vi "Configure Dialog.vi"(8 "error in (no error)":errorcluster, 11 "Configure AM Internal [AM] Msg.lvclass":refnum<class "Configure AM Internal [AM] Msg.lvclass">) -> (0 "error out":errorcluster, 2 "Ok?":bool, 3 "Configure AM Internal [AM] Msg.lvclass":refnum<class "Configure AM Internal [AM] Msg.lvclass">)   [LabVIEW 2015, in "CS++Fgen.lvlib" / "Configure AM Internal [AM] Msg.lvclass"]
uses:
  Configure AM Internal [AM] Msg.lvclass
  Configure AM Internal [AM] Msg.lvclass/Configure AM Internal [AM] Msg.ctl
panel:
  in  "modulation waveform (Sine)":i32
  in  "Cancel Button":bool
  in  "OK Button":bool
  in  "modulation frequency":dbl[unit]
  in  "modulation depth":dbl
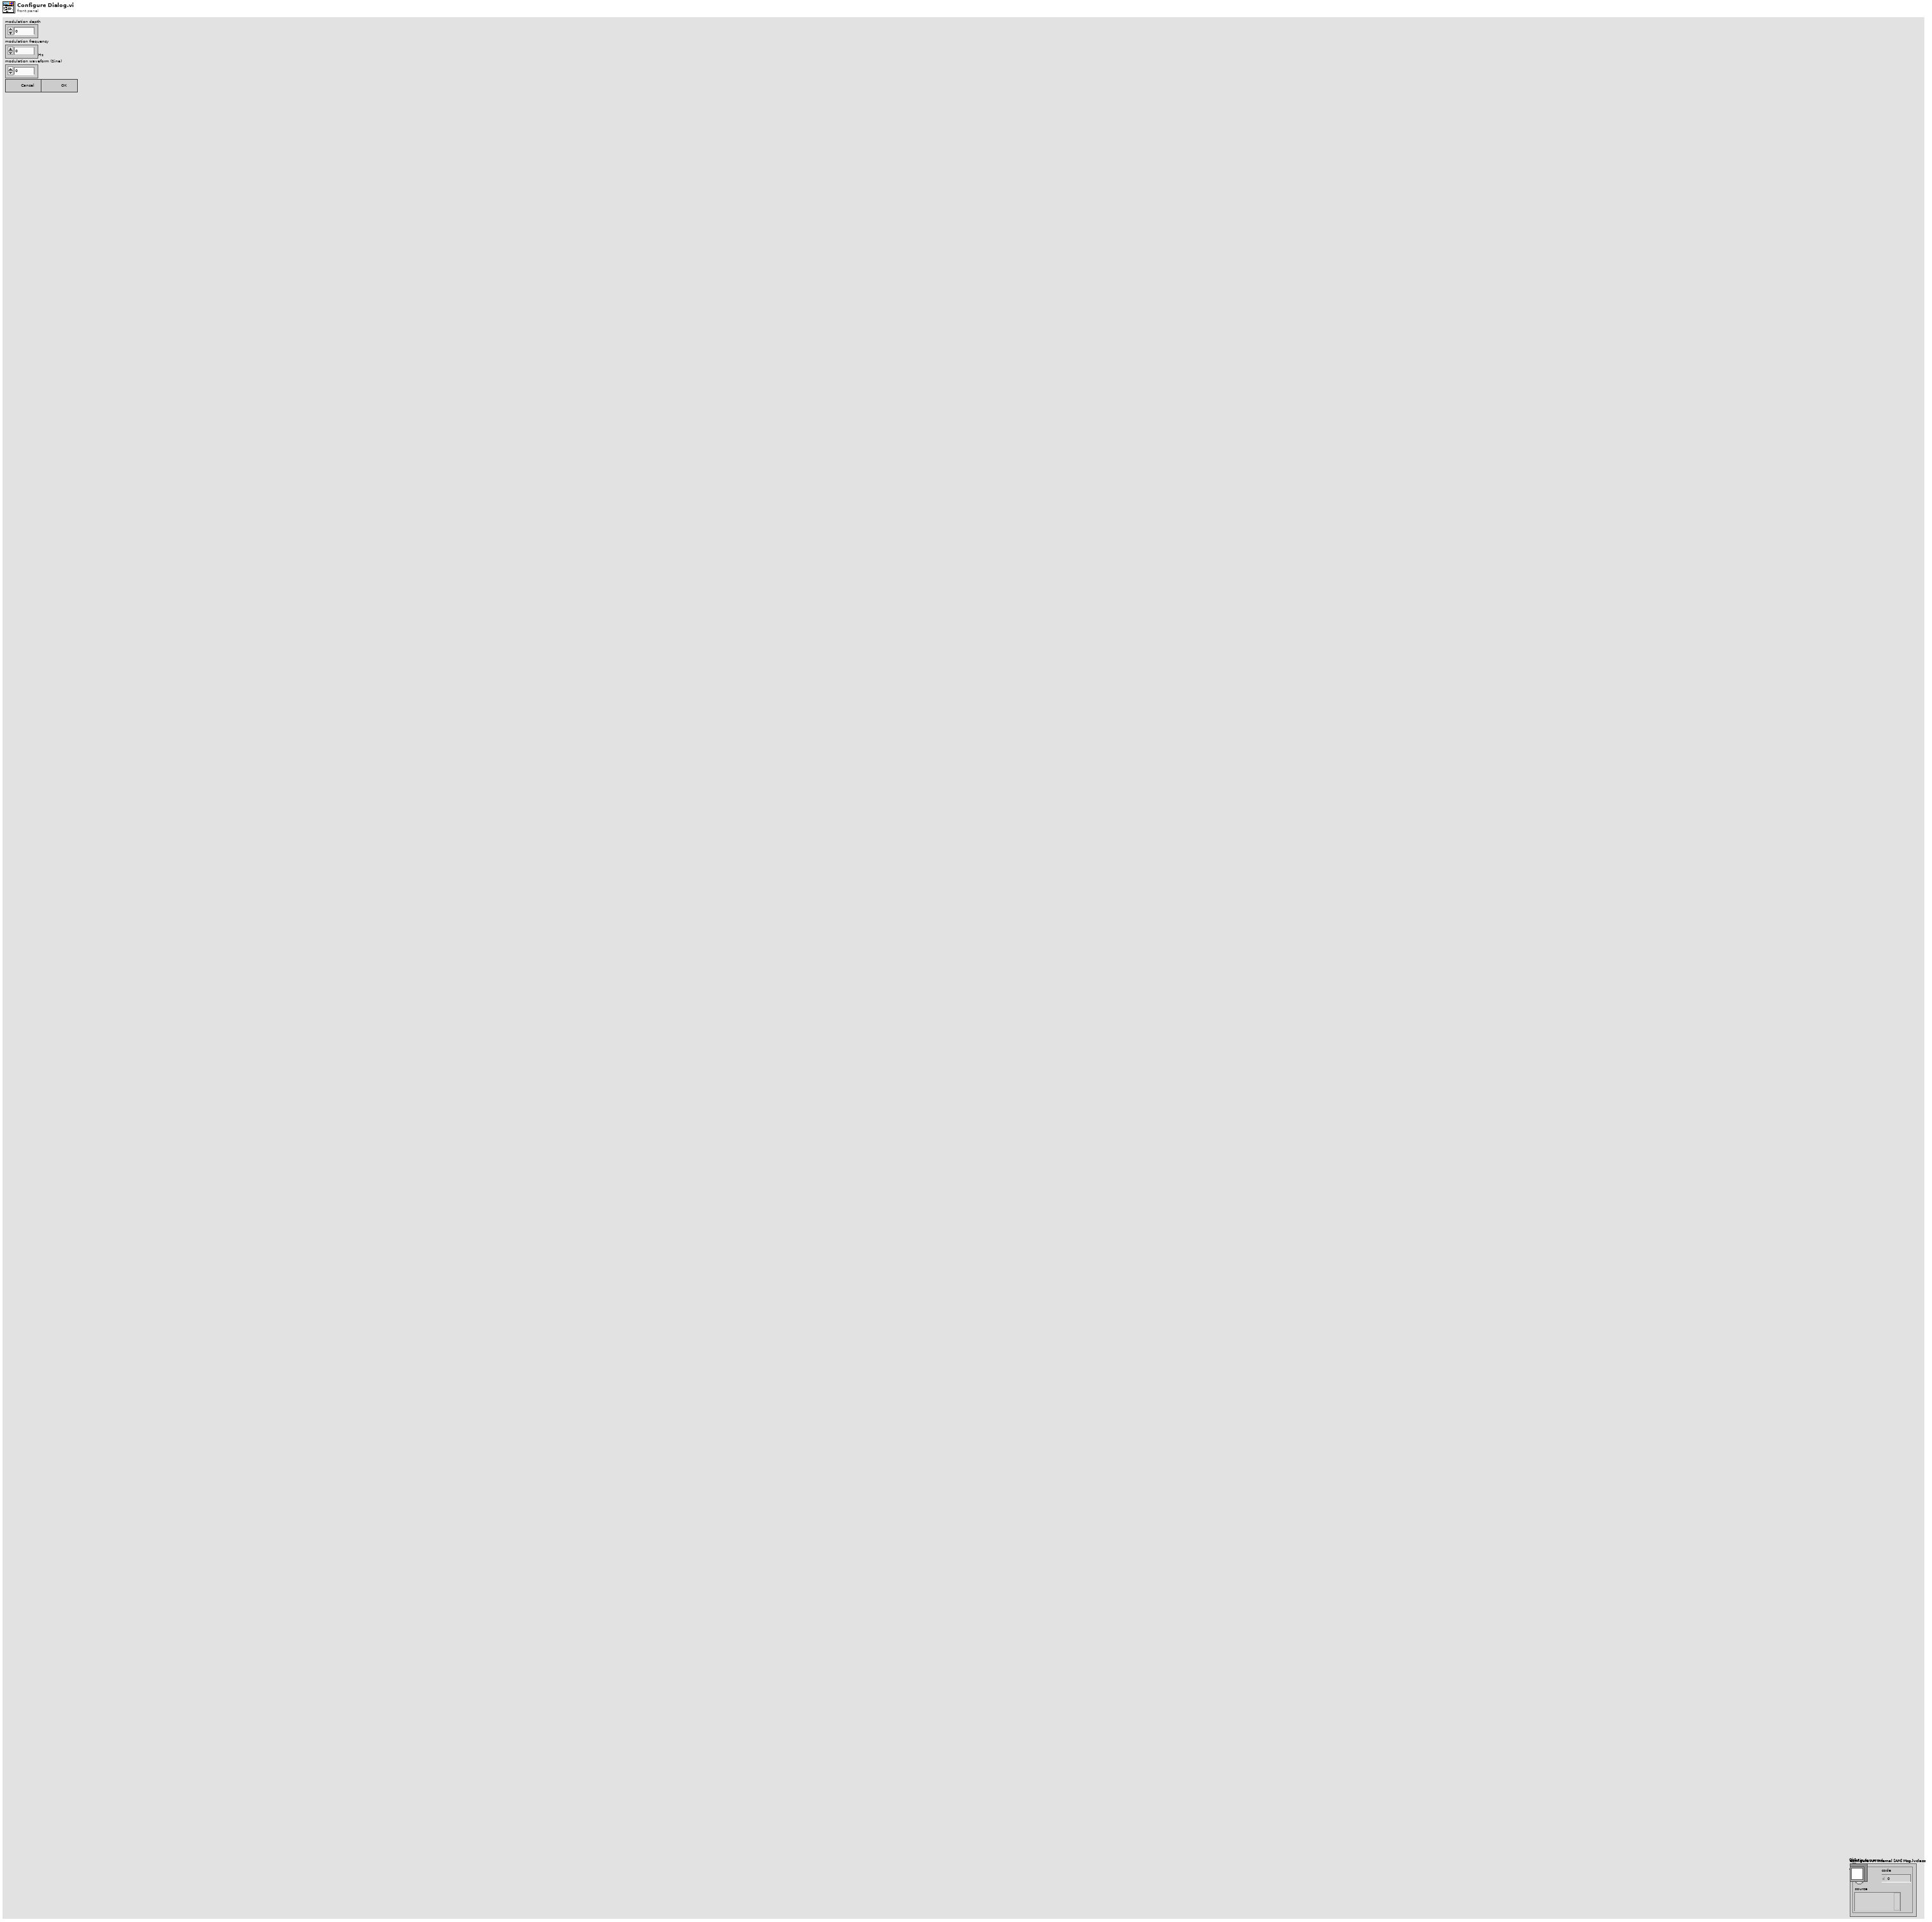
[diagram p1: front panel]
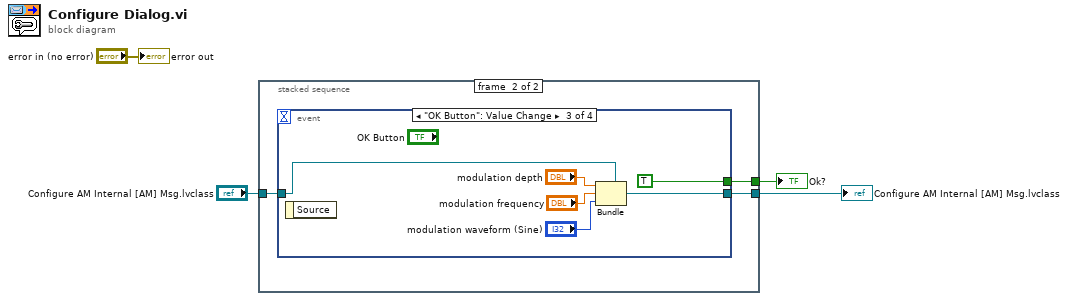
[diagram p0: block diagram]
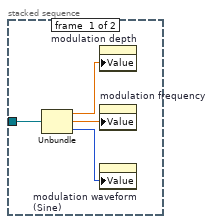
[diagram p2: hidden frame]
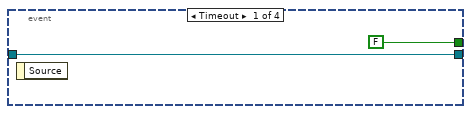
[diagram p3: hidden frame]
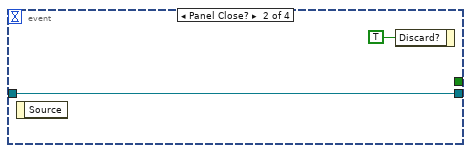
[diagram p4: hidden frame]
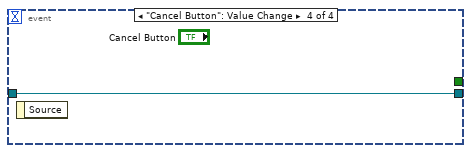
[diagram p5: hidden frame]
diagram:
  n1 = stacked-sequence {
    tunnel: [_ w11] -> w3
    tunnel: [_ w10] -> w2
    tunnel: "Configure AM Internal [AM] Msg.lvclass" -> [w8 w9]
    frame #0 {
      n2 = Unbundle ("Seq0Unbundler")(w8) -> (w7:dbl, w6:dbl[unit], w5:i32)
      n3 = property on="modulation depth" class="DigNum (strict)"("Value"=w7) -> ()  [unwired: 2 in, 2 out]
      n4 = property on="modulation frequency" class="DigNum (strict)"("Value"=w6) -> ()  [unwired: 2 in, 2 out]
      n5 = property on="modulation waveform (Sine)" class="DigNum (strict)"("Value"=w5) -> ()  [unwired: 2 in, 2 out]
    }
    frame #1 {
      n6 = event shown="[2] \"OK Button\": Value Change" {
        selector: _ -> [_ _ _ _]
        dyn-events: _ -> [_ _ _ _]
        timeout: _ -> [_ _ _ _]
        tunnel: [w12 w14 w19 w22] -> w10
        tunnel: w9 -> [w12 w14 w21 w22]
        tunnel: [FALSE _ TRUE _] -> w11
        event Timeout {
          n7 = event-data() -> ()  [unwired: 1 in, 1 out]
        }
        event Panel Close? {
          n8 = event-data() -> ()  [unwired: 1 in, 1 out]
          n9 = event-data ("Event Filter Node")("Discard?"=TRUE) -> ()  [unwired: 1 in, 1 out]
        }
        event "OK Button": Value Change {
          n10 = event-data() -> ()  [unwired: 1 in, 1 out]
          n11 = Bundle ("Main-Bundler")(cluster=w21, "modulation depth", "modulation frequency", "modulation waveform (Sine)") -> (w19:refnum<class "Configure AM Internal [AM] Msg.lvclass">)
        }
        event "Cancel Button": Value Change {
          n12 = event-data() -> ()  [unwired: 1 in, 1 out]
        }
      }
    }
  }
  "Ok?" <- w3
  "Configure AM Internal [AM] Msg.lvclass" <- w2
  "error out" <- "error in (no error)"
